vi "Set_shutdown_HV.vi"() -> ()   [LabVIEW 2012]
uses:
  hv cluster control.ctl
  <vilib>/Platform/TimedLoop/XDataNode/timing_clust.ctl
  <vilib>/Platform/TimedLoop/XDataNode/nitl_modes.ctl
  <vilib>/Platform/TimedLoop/XDataNode/wakeup.ctl
  <vilib>/Platform/TimedLoop/XDataNode/XDataNode.xnode
  CAEN/labview/CAENHVWrapper/CAENHVWrapper.lvlib
  <vilib>/Platform/TimedLoop/XDataNode/XDNodeRunTimeDep.lvlib
panel:
  out "retval":i32
  out "error out":errorcluster
  in  "stop":bool
  in  "Set the HVs?":bool
  in  "HV Power On/Off":bool[](array[boolean])=[TRUE, TRUE, FALSE, FALSE, FALSE, FALSE, FALSE, FALSE]
  in  "HV Tolerance (%)":dbl=1.0
  in  "Set Voltage":string[](array[string])=["100", "0", "0", "0", "0", "0", "0", "0"]
  out "handle":i32
  in  "IP adress HV2":string="1_0_0"
  in  "IP adress HV1":string="0_0_0"
  in  "HV Cluster":T1={"HV Power On/Off"=[TRUE, TRUE], "Set Voltage"=["0", "0", "0", "0", "0", "0", "0", "0"], "HV Tolerance (%)"=1.0}
  # "Turn off HVs"
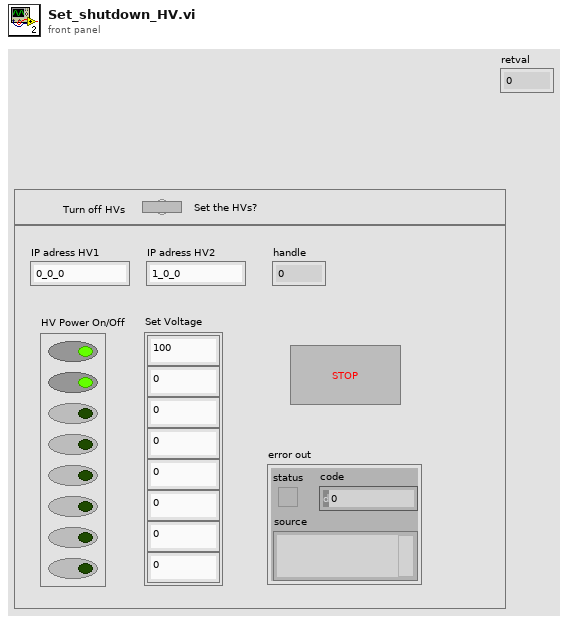
[diagram p1: front panel]
types:
  T1 = typedef "hv cluster control.ctl" = cluster{"HV Power On/Off":bool[], "Set Voltage":string[], "HV Tolerance (%)":dbl}
  T2 = typedef "XDNodeRunTimeDep.lvlib/timing_clust.ctl" = cluster{"Expected End [f-1]":u64, "Actual End [f-1]":u64, "Finished Late? [f-1]":bool, "Expected End [i-1]":u64, "Actual End [i-1]":u64, "Finished Late? [i-1]":bool, "Expected Start [i]":u64, "Actual Start [i]":u64, "Expected Start [f]":u64, "Actual Start [f]":u64, "Source Name":string, "Structure Name":string, "Period":i64, "Deadline":i64, "Offset":i64, "Start":i64, "Priority":i32, "Timeout":i32, "Mode":T3, "Wakeup Reason":T4, "Error":errorcluster, "Source Type":string, "Secondary Source Type":string, "Global End Time":u64, "Global Start Time":u64, "Frame Duration":u64, "Iteration Duration":u64, "Assigned CPU":i32, "I/O Scan Engine Mode":u32}
  T3 = typedef "XDNodeRunTimeDep.lvlib/nitl_modes.ctl" = enum32{"No Change", "Process missed periods, maintain original phase", "Discard missed periods, maintain original phase", "Process missed periods, ignore original phase", "Discard missed periods, ignore original phase"}
  T4 = typedef "XDNodeRunTimeDep.lvlib/wakeup.ctl" = enum32{"Normal", "Aborted", "Asynchronous wakeup", "Timing source error", "Timed loop error", "Timeout"}
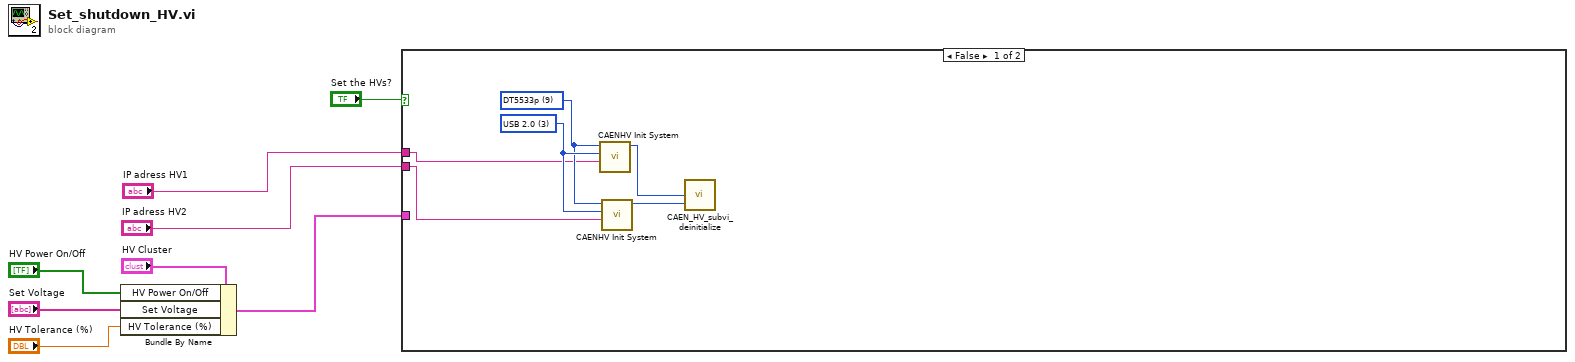
[diagram p0: block diagram]
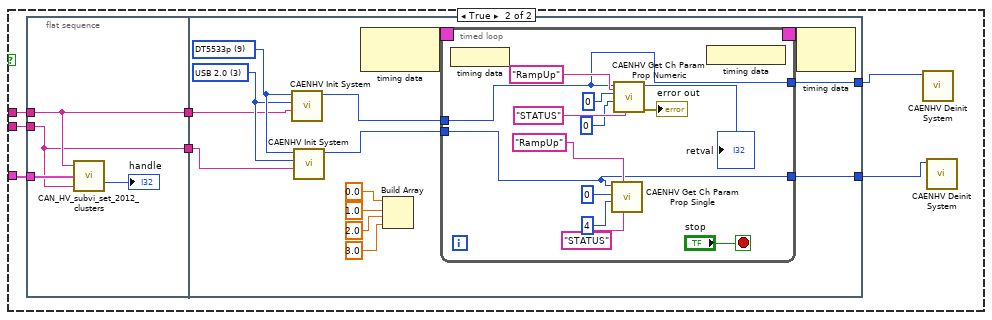
[diagram p2: hidden frame]
diagram:
  n1 = Bundle By Name(cluster="HV Cluster", "HV Power On/Off"="HV Power On/Off", "Set Voltage"="Set Voltage", "HV Tolerance (%)"="HV Tolerance (%)") -> (w4:T1)
  n2 = case shown="False" "Set the HVs?" {
    tunnel: "IP adress HV1" -> [w10 w20]
    tunnel: "IP adress HV2" -> [w9 w19]
    tunnel: w4 -> [_ w21]
    frame False {
      w14 = 3 items=["TCP/IP"=0, "HS CAENET"=2, "USB 2.0"=3, "CONET Optical Link"=4, "USB VCP"=5] ("LinkType")
      w13 = u32 9 items=["SY1527", "SY2527", "SY4527", "SY5527", "N568", "V65XX", "N1470", "V8100", "", "DT5533p"] ("system")
      n3 = call "CAENHV Init System.vi"("Arg"=w10, "LinkType"=w14, "system"=w13) -> ("handle"=w11:i32)  [unwired: 7 in, 1 out]
      n4 = call "CAENHV Init System.vi"("Arg"=w9, "LinkType"=w14, "system"=w13) -> ("handle"=w12:i32)  [unwired: 7 in, 1 out]
      n5 = call "CAEN_HV_subvi_deinitialize.vi"("Handle 2"=w12, "Handle 1"=w11) -> ()  [unwired: 1 in, 1 out]
    }
    frame True {
      n6 = flat-sequence {
        tunnel: w21 -> [w24]
        tunnel: w20 -> [w23]
        tunnel: w19 -> [w22]
        tunnel: [w23] -> w18
        tunnel: [w22] -> w17
        tunnel: w18 -> [w29]
        tunnel: w17 -> [w28]
        tunnel: [w27] -> w16
        tunnel: [w26] -> w15
        frame #0 {
          n7 = call "CAN_HV_subvi_set_2012_clusters.vi"("IP adress HV2"=w22, "HV Cluster"=w24, "IP adress HV1"=w23) -> ("handle"=→"handle":i32)  [unwired: 1 out]
        }
        frame #1 {
          w30 = 3 items=["TCP/IP"=0, "HS CAENET"=2, "USB 2.0"=3, "CONET Optical Link"=4, "USB VCP"=5] ("LinkType")
          w31 = u32 9 items=["SY1527", "SY2527", "SY4527", "SY5527", "N568", "V65XX", "N1470", "V8100", "", "DT5533p"] ("system")
          n8 = call "CAENHV Init System.vi"("Arg"=w29, "LinkType"=w30, "system"=w31) -> ("handle"=w32:i32)  [unwired: 7 in, 1 out]
          n9 = call "CAENHV Init System.vi"("Arg"=w28, "LinkType"=w30, "system"=w31) -> ("handle"=w33:i32)  [unwired: 7 in, 1 out]
          n10 = node-c288() -> (w39:T2)  [unwired: 1 in]
          n11 = Build Array(0.0 ("element"), 1.0 ("element"), 2.0 ("element"), 3.0 ("element")) -> ()  [unwired: 1 out]
          n12 = timed-loop {
            timing: w39 -> [_]
            timing-out: [_] -> w38
            tunnel: w32 -> [w44]
            tunnel: w33 -> [w43]
            tunnel: [w44] -> w27
            tunnel: [w43] -> w26
            stop <- "stop" stop-if-true
            n13 = node-c288() -> ()  [unwired: 1 in]
            n14 = call "CAENHV Get Ch Param Prop Single.vi"("PropName"="STATUS", "ParName"="RampUp", "Ch"=u16 4 ("ChNum (1)"), "slot"=u16 0 ("Ch"), "handle"=w43) -> ()  [unwired: 5 in, 2 out]
            n15 = call "CAENHV Get Ch Param Prop Numeric.vi"("PropName"="STATUS", "ParName"="RampUp", "Ch"=u16 0 ("ChNum (1)"), "slot"=u16 0 ("Ch"), "handle"=w44) -> ("error out"=→"error out":errorcluster, "retval"=→"retval":i32)  [unwired: 5 in]
            n16 = node-c288() -> ()  [unwired: 1 out]
          }
          n17 = node-c288(w38) -> ()  [unwired: 1 out]
        }
      }
      n18 = call "CAENHV Deinit System.vi"("handle"=w16) -> ()  [unwired: 10 in, 1 out]
      n19 = call "CAENHV Deinit System.vi"("handle"=w15) -> ()  [unwired: 10 in, 1 out]
    }
  }
